vi "CalcRobotDeltaHeading.vi"(2 "New Rate of Turn":dbl, 3 "New Robot Heading":dbl, 8 "Previous Rate of Turn":dbl, 9 "Rudder Position":dbl, 10 "Sail Position":dbl, 11 "Old Robot Heading":dbl) -> ()   [LabVIEW 2012]
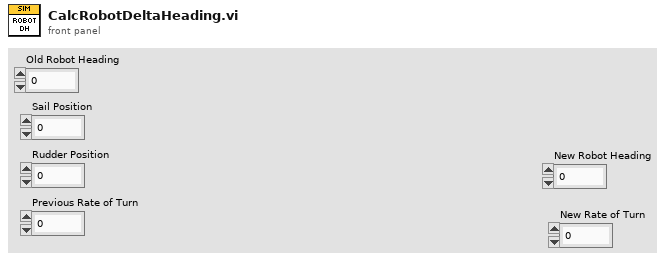
[diagram p1: front panel]
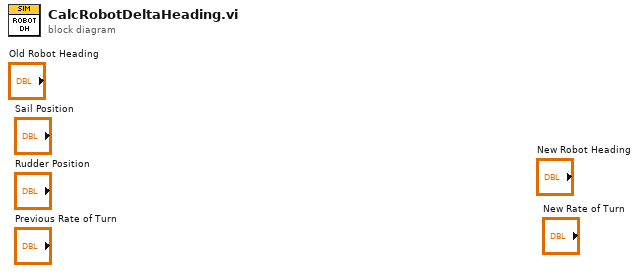
[diagram p0: block diagram]
diagram:
